vi "Get Base Command.vi"(8 "error in (no error)":errorcluster, 11 "Output in":refnum<class "Output.lvclass">) -> (0 "error out":errorcluster, 2 "Base Command":string, 3 "Output out":refnum<class "Output.lvclass">)   [LabVIEW 2023, in "HAF.lvlib" / "Output.lvclass"]
doc: "Returns the base command whch is used to build up the overall command string – parameters will be added to this as necessary.  The framework will add the line terminator \\n.\n\nSubclasses MUST override this member and must not add a line terminator on the end of the command; on this class an error is returned."
uses:
  Output.lvclass
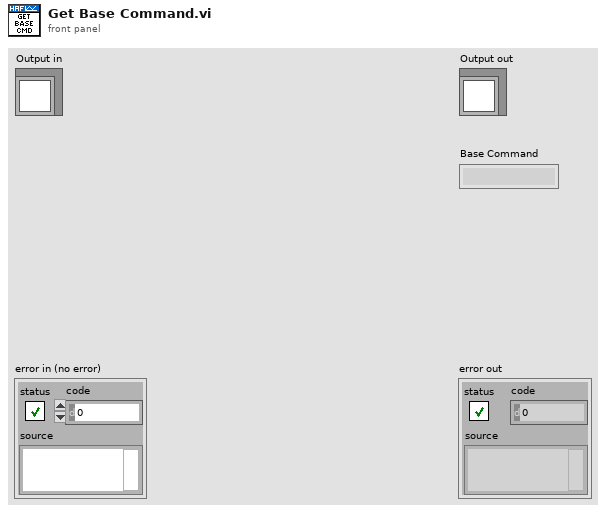
[diagram p1: front panel]
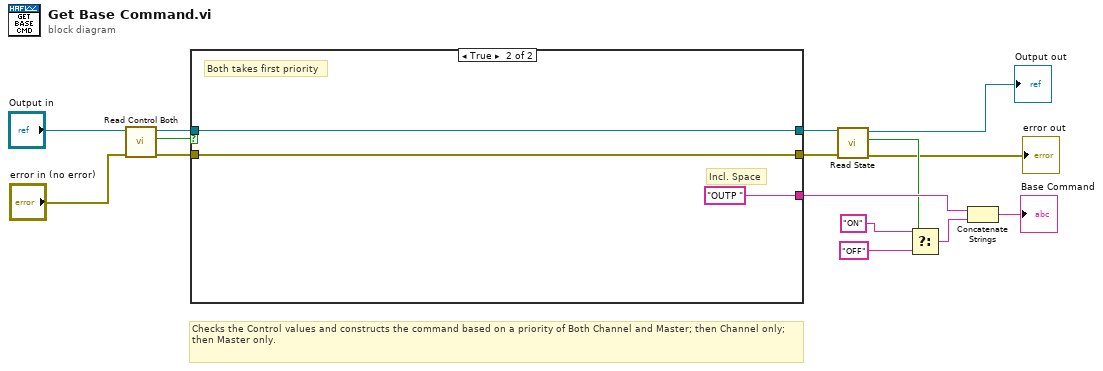
[diagram p0: block diagram]
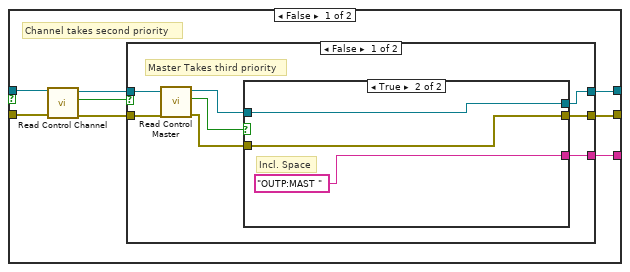
[diagram p2: hidden frame]
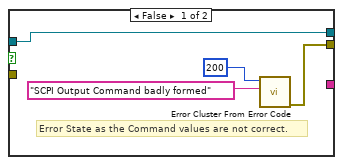
[diagram p3: hidden frame]
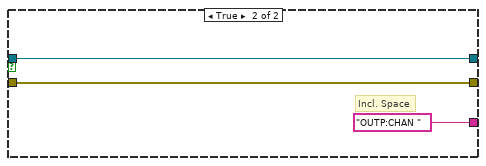
[diagram p4: hidden frame]
diagram:
  # "Checks the Control values and constructs the command based on a priority of Both Channel and Master; then Channel only; then Master only."
  n1 = call-dynamic "Read Control Both.vi"("error in (no error)"="error in (no error)", "Output in"="Output in") -> ("error out"=w11:errorcluster, "Control Both"=w13:bool, "Output out"=w12:refnum<class "Output.lvclass">)  [unwired: 7 in]
  n2 = case shown="True" w13 {
    tunnel: w12 -> [w23 w42]
    tunnel: w11 -> [w22 w43]
    tunnel: [w16 "OUTP "] -> w10
    tunnel: [w17 w43] -> w8
    tunnel: [w18 w42] -> w9
    frame False {
      # "Channel takes second priority"
      n3 = call-dynamic "Read Control Channel.vi"("error in (no error)"=w22, "Output in"=w23) -> ("error out"=w19:errorcluster, "Control Channel"=w21:bool, "Output out"=w20:refnum<class "Output.lvclass">)  [unwired: 7 in]
      n4 = case shown="False" w21 {
        tunnel: w20 -> [w31 w41]
        tunnel: w19 -> [w30 w40]
        tunnel: [w24 w41] -> w18
        tunnel: [w25 w40] -> w17
        tunnel: [w26 "OUTP:CHAN "] -> w16
        frame False {
          # "Master Takes third priority"
          n5 = call-dynamic "Read Control Master.vi"("error in (no error)"=w30, "Output in"=w31) -> ("error out"=w27:errorcluster, "Control Master"=w29:bool, "Output out"=w28:refnum<class "Output.lvclass">)  [unwired: 7 in]
          n6 = case shown="True" w29 {
            tunnel: w28 -> [w35 w36]
            tunnel: w27 -> [_ w37]
            tunnel: [_ "OUTP:MAST "] -> w26
            tunnel: [w32 w37] -> w25
            tunnel: [w35 w36] -> w24
            frame False {
              # "Error State as the Command values are not correct."
              n7 = call <vilib>:"Error Cluster From Error Code.vi"("error message (\"\")"="SCPI Output Command badly formed" ("error message (\"\")"), "error code (0)"=200) -> ("error out"=w32:errorcluster)  [unwired: 7 in]
            }
            frame True {
              # "Incl. Space"
            }
          }
        }
        frame True {
          # "Incl. Space"
        }
      }
    }
    frame True {
      # "Both takes first priority"
      # "Incl. Space"
    }
  }
  n8 = call-dynamic "Read State.vi"("error in (no error)"=w8, "Output in"=w9) -> ("error out"=→"error out":errorcluster, "State"=w7:bool, "Output out"=→"Output out":refnum<class "Output.lvclass">)  [unwired: 7 in]
  n9 = Select(t="ON", s=w7, f="OFF") -> (s? t:f=w4:string)
  n10 = Concatenate Strings(w10, w4) -> (→"Base Command":string)
